vi "Tree selection FGV LUT.vi"(10 "Ref":refnum<vi>, 11 "Loop data":T1[](array[typedef])) -> (1 "Index":i32, 2 "Ref (dup)":refnum<vi>, 3 "Loop data":T1[](array[typedef]))   [LabVIEW 2020, in "UI_ItemSelect_OpenSource.lvlib"]
uses:
  UI_ItemSelect_OpenSource.lvlib
  Tree item select loop data.ctl
  Item select ref type.ctl
  Tree item loop data.ctl
  Tree item selection indices.ctl
  checkbox state.ctl
  item select tree lock states.ctl
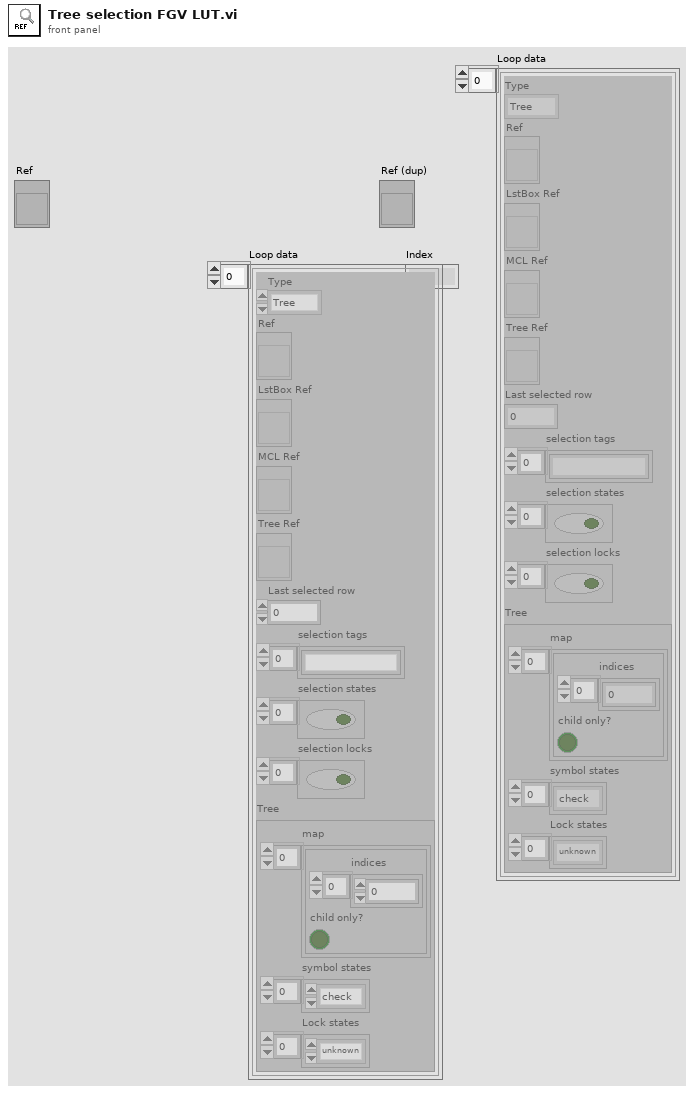
[diagram p1: front panel]
types:
  T1 = typedef "UI_ItemSelect_OpenSource.lvlib/Tree item select loop data.ctl" = cluster{"Type":T2, "Ref":refnum<vi>, "LstBox Ref":refnum<vi>, "MCL Ref":refnum<vi>, "Tree Ref":refnum<vi>, "Last selected row":i32, "selection tags":string[], "selection states":bool[], "selection locks":bool[], "Tree":T3}
  T2 = typedef "UI_ItemSelect_OpenSource.lvlib/Item select ref type.ctl" = enum16{"Tree", "MCL", "ListBox"}
  T3 = typedef "UI_ItemSelect_OpenSource.lvlib/Tree item loop data.ctl" = cluster{"map":T4[], "symbol states":T5[], "Lock states":T6[]}
  T4 = typedef "UI_ItemSelect_OpenSource.lvlib/Tree item selection indices.ctl" = cluster{"indices":i32[], "child only?":bool}
  T5 = typedef "UI_ItemSelect_OpenSource.lvlib/checkbox state.ctl" = enum16{"unknown", "check", "some", "no check"}
  T6 = typedef "UI_ItemSelect_OpenSource.lvlib/item select tree lock states.ctl" = enum16{"unknown", "locked", "unlocked"}
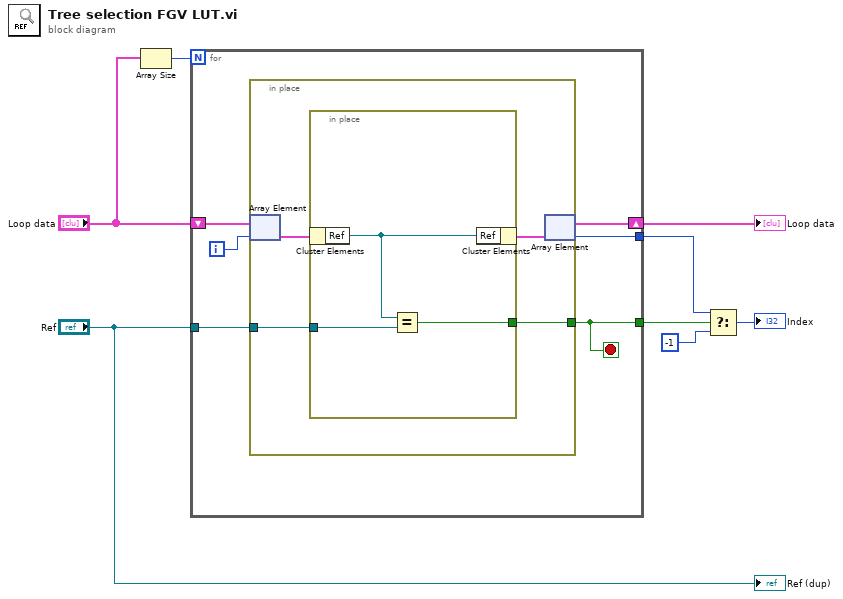
[diagram p0: block diagram]
diagram:
  n1 = Array Size(array="Loop data") -> (size(s)=w8:i32)
  n2 = for {
    N: w8 -> [_]
    shift-right: [w11] -> w1
    shift-left: "Loop data" -> [w14]
    tunnel: "Ref" -> [w12]
    tunnel: [w10] -> w4
    tunnel: [w9] -> w5
    i -> [w13]
    stop <- w9 stop-if-true
    n3 = in-place {
      in-place-border: w12 -> [w17]
      in-place-border: [w15] -> w9
      n4 = in-place-array #1(w14, w13) -> (w18:T1)
      n5 = in-place {
        in-place-border: w17 -> [w20]
        in-place-border: [w19] -> w15
        n6 = in-place-cluster #2(w18) -> ("Ref"=w21:refnum<vi>)
        n7 = Equal?(x=w21, y=w20) -> (x = y?=w19:bool)
        n8 = in-place-cluster #2("Ref"=w21) -> (w16:T1)
      }
      n9 = in-place-array #1(w16) -> (w11:T1[], w10:i32)
    }
  }
  "Loop data" <- w1
  n10 = Select(t=w4, s=w5, f=-1) -> (s? t:f=→"Index":i32)
  "Ref (dup)" <- "Ref"
